vi "数组案例之空字符串去除.vi"() -> ()   [LabVIEW 2018]
panel:
  out "数组 2":string[](array[string])
  in  "数组":string[](array[string])
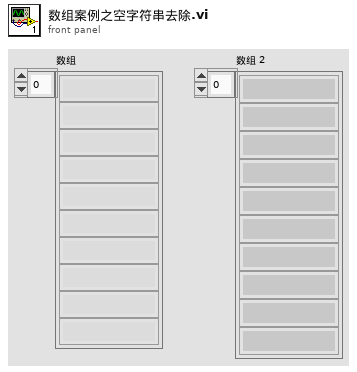
[diagram p1: front panel]
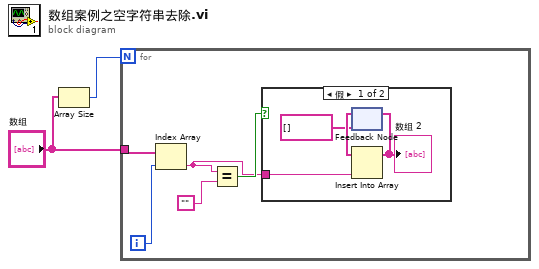
[diagram p0: block diagram]
diagram:
  n1 = Array Size(array="数组") -> (size(s)=w1:i32)
  n2 = for {
    N: w1 -> [_]
    tunnel: "数组" -> [w7]
    i -> [w6]
    n3 = Index Array(array=w7, index=w6) -> (element=w3:string)
    n4 = Equal?(x=w3, y="") -> (x = y?=w4:bool)
    n5 = case shown="假" w4 {
      tunnel: w3 -> [w11 _]
      frame False {
        n6 = feedback #1(string[] []) -> (w9:string[])
        n7 = Insert Into Array(array=w9, new element=w11) -> (w10:string[])  [unwired: 1 in]
        "数组 2" <- w10
        n8 = feedback-in #1(w10) -> ()
      }
      frame True {
      }
    }
  }
